vi "displacementTest.vi"   [LabVIEW 2016]
uses:
  FPGAMockDisplacement/DataTypes/MockDisplacementSettings.ctl
  Common_FPGA_SerialASCII/DataTypes/SerialASCIISettings.ctl
  FPGAMockDisplacement/FPGAMockDisplacement.lvlib
  Common_FPGA_SerialASCII/FPGASerialASCII.lvlib
types:
  T1 = typedef "FPGASerialASCII.lvlib/SerialASCIISettings.ctl" = cluster{"SerialPort":refnum<k21>, "TimestampRegister":refnum<k21>, "TxFIFO":refnum<k21>, "RxFIFO":refnum<k21>, "Terminator":u8, "ReadTimeoutMs":i16, "IRQ":u8}
  T2 = typedef "FPGAMockDisplacement.lvlib/MockDisplacementSettings.ctl" = cluster{"SerialPort":refnum<k21>, "BufferUpdateFIFO":refnum<k21>, "DisplacementMemory":refnum<k21>}
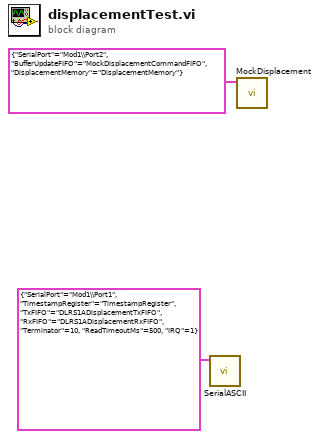
[diagram p0: block diagram]
diagram:
  n1 = call "SerialASCII.vi"("SerialASCIISettings"=T1 {"SerialPort"="Mod1\\Port1", "TimestampRegister"="TimestampRegister", "TxFIFO"="DLRS1ADisplacementTxFIFO", "RxFIFO"="DLRS1ADisplacementRxFIFO", "Terminator"=10, "ReadTimeoutMs"=500, "IRQ"=1}) -> ()  [unwired: 11 in]
  n2 = call "MockDisplacement.vi"("MockDisplacementSettings"=T2 {"SerialPort"="Mod1\\Port2", "BufferUpdateFIFO"="MockDisplacementCommandFIFO", "DisplacementMemory"="DisplacementMemory"}) -> ()  [unwired: 11 in]
